vi "ChipKit Continuous Sampling.vi"() -> ()   [LabVIEW 2011, in "LabVIEW Interface for ChipKit.lvlib"]
doc: "This VI shows an example of using the continuous aquisition mode on the ChipKit to aquire analog input data from a single input pin. The user can set the sample rate for the aquisition when the VI is first run. The maximum aquisition speed of the ChipKit is 5KHZ. While this mode is turned on executing other LIFCK commands will corrupt analog data. To use other LIFCK commands turn continuous mode off first."
uses:
  vi.lib/LabVIEW Interface for ChipKit/LabVIEW Interface for ChipKit.lvlib
panel:
  in  "VISA resource name":refnum<visa-resource-name>
  out "Waveform Chart":dbl[](graph)
  in  "Stop":bool
  in  "Sample Rate (HZ)":u16
  in  "Analog Input Pin":u8
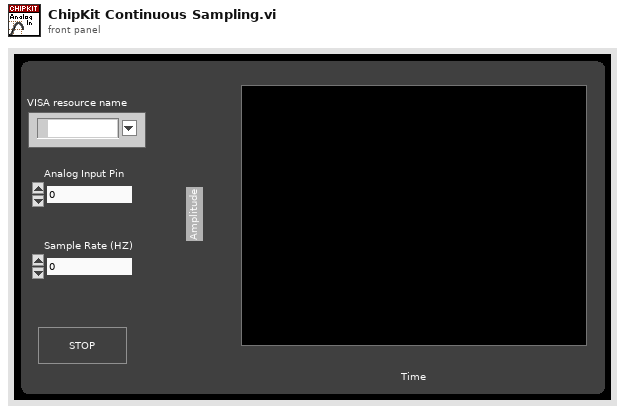
[diagram p1: front panel]
types:
  T1 = typedef "LabVIEW Interface for ChipKit.lvlib/Chipkit Resource.ctl" = cluster{"VISA resource":refnum<visa-resource-name>, "Board Type":T2, "Connection Type":enum8{"USB / Serial"}, "Bytes Per Packet (15)":u8}
  T2 = typedef "LabVIEW Interface for ChipKit.lvlib/Board Type.ctl" = enum16{"Arduino Uno", "Dimuelanove w/Atmega 328", "Mega 2560", "Chipkit Uno32", "Chipkit Max32"}
  T3 = typedef "LabVIEW Interface for ChipKit.lvlib/Chipkit Resource.ctl" = cluster{"COM Port":refnum<visa-resource-name>, "Board Type":T4, "Connection Type":T5, "Baud Rate (115200)":u32, "Bytes Per Packet (15)":u32}
  T4 = typedef "LabVIEW Interface for ChipKit.lvlib/Board Type.ctl" = enum16{"ChipKit uC32", "ChipKit Uno32", "ChipKit Max32"}
  T5 = typedef "LabVIEW Interface for ChipKit.lvlib/Connection Type.ctl" = enum8{"USB / Serial", "XBEE", "BlueSmirf (Bluetooth)"}
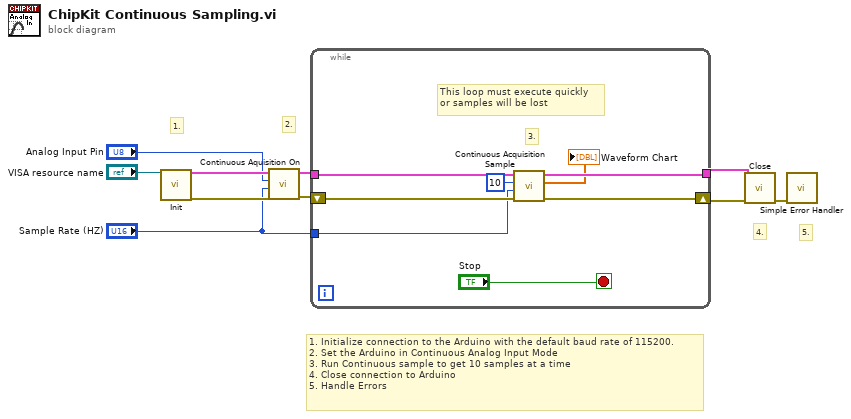
[diagram p0: block diagram]
diagram:
  # "5."
  # "4."
  # "2."
  # "1."
  # "1. Initialize connection to the Arduino with the default baud rate of 115200.\n2. Set the Arduino in Continuous Analog Input Mode\n3. Run Continuous sample to get 10 samples at a time\n4. Close connection to Arduino\n5. Handle Errors"
  n1 = call "Init.vi"("VISA resource"="VISA resource name") -> ("Arduino Resource"=w10:T1, "error out"=w3:errorcluster)  [unwired: 17 in]
  n2 = call "Continuous Aquisition On.vi"("error in"=w3, "Acquition Speed"="Sample Rate (HZ)", "Analog Input Pin"="Analog Input Pin", "Arduino Resource"=w10) -> ("error out"=w8:errorcluster, "Arduino Resource"=w9:T3)  [unwired: 6 in]
  n3 = while {
    tunnel: w9 -> [w17]
    tunnel: [w16] -> w7
    shift-right: [w15] -> w4
    shift-left: w8 -> [w14]
    tunnel: "Sample Rate (HZ)" -> [w11]
    stop <- "Stop" stop-if-true
    # "This loop must execute quickly\nor samples will be lost"
    # "3."
    n4 = call "Continuous Acquisition Sample.vi"("Arduino Resource"=w17, "Samples to Read"=u16 10, "Sample Rate (HZ)"=w11, "error in (no error)"=w14) -> ("Arduino Resource"=w16:T3, "Data"=→"Waveform Chart":dbl[], "error out"=w15:errorcluster)  [unwired: 4 in]
  }
  n5 = call "Close.vi"("Arduino Resource"=w7, "error in"=w4) -> ("error out"=w6:errorcluster)  [unwired: 13 in]
  n6 = call <vilib>:"Simple Error Handler.vi"("error in (no error)"=w6) -> ()  [unwired: 4 in, 5 out]
